vi "Launch uService.vi"(4 "Highlander?":bool, 6 "uService ID":string, 8 "error in (no error)":errorcluster, 9 "GUI?":bool, 10 "uService Class Name":string, 11 "Guardian in":refnum<class "Guardian.lvclass">) -> (0 "error out":errorcluster, 3 "Guardian out":refnum<class "Guardian.lvclass">)   [LabVIEW 2026, in "TALOS.lvlib" / "Guardian.lvlib" / "Guardian.lvclass"]
doc: "This VI get called everytime a uService has to be launched. The optional uService ID input is needed if a different name is wanted for a specific uService, otherwise the class name is used (useful when launching more than an instance of a uService, for example)."
uses:
  Guardian.lvclass
  C:/LabVIEW Code/TALOS/talos/Ancestor/Ancestor/Ancestor.lvclass
  C:/LabVIEW Code/TALOS/builds/Actor Framework PPL/Actor Framework.lvlibp/1abvi3w/vi.lib/ActorFramework/Actor/Actor.lvclass
  Classes/uService List/uService Properties.ctl
  builds/Actor Framework PPL/Actor Framework.lvlibp/1abvi3w/vi.lib/ActorFramework/Message Enqueuer/Message Enqueuer.lvclass
  Ancestor/Ancestor/Ancestor.lvclass/Ancestor.ctl
  Classes/uService List/uService List.lvclass/uService List.ctl
  Guardian Messages/Broadcast to Guardians Msg/Broadcast to Guardians Msg.lvclass/Broadcast to Guardians Msg.ctl
  Guardian.lvclass/Guardian.ctl
  Ancestor/Ancestor/Write Distr uS Map ref.vi
  Ancestor/Ancestor/Read ID.vi
  Ancestor/Ancestor/Read Distr uS Map ref.vi
  Support VIs/Generate Error.vi
  FGV/Error Memory/Get Error Description.vi
  Support VIs/Get PC name.vi
  Support VIs/Get Class Name.vi
  <vilib>/Utility/error.llb/Clear Errors.vi
  FGV/Error Memory/Error Memory Core.vi
  <vilib>/AdvancedString/Delimited String to 1D String Array.vi
  <vilib>/AdvancedString/Delimited String to 1D String Array (string).vi
  Support VIs/Circus Root Path.vi
  FGV/Error Memory/Error Crt Lvl checker.vi
  FGV/Error Memory/Error Memory Core.vi/40c8088d-b597-4017-91af-faa98e00292e.vi
  FGV/Error Memory/Error Memory Core.vi/d4a3ab98-063c-4e44-b43d-fbdcfe6c2be2.vi
  Father of all uServices/Father of all uServices/Father of all uServices.lvclass
  builds/Actor Framework PPL/Actor Framework.lvlibp/1abvi3w/vi.lib/ActorFramework/Message Enqueuer/Enqueue.vi
  Support VIs/Global Memory.vi
  <vilib>/Utility/LVClass/Get LV Class Name.vi
  Support VIs/Is in Packed Library.vi
  Support VIs/TALOS Root path.vi
  Support VIs/Read CSV worksheet.vi
  Support VIs/Global Constants.vi
  <vilib>/Utility/error.llb/General Error Handler.vi
  Support VIs/Error Log.vi
  Classes/Distributed uService Map/Distributed uService Map.lvclass
  Classes/uService List/uService List.lvclass
  Guardian Messages/Broadcast to Guardians Msg/Broadcast to Guardians Msg.lvclass
  Ancestor/Ancestor/Ancestor.lvclass
  <vilib>/Comparison/Equal/Equal Functor/Equal Functor.lvclass
  builds/Actor Framework PPL/Actor Framework.lvlibp/1abvi3w/vi.lib/ActorFramework/Actor/Actor.lvclass
  TALOS.lvlib
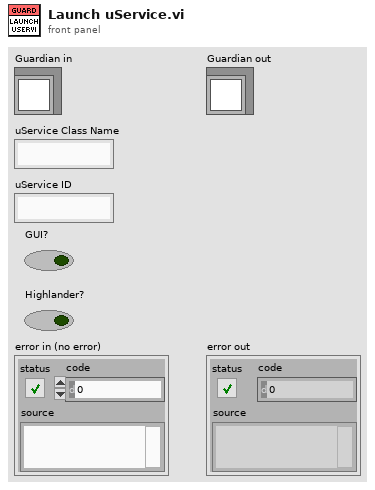
[diagram p1: front panel]
types:
  T1 = typedef "TALOS.lvlib/Classes.lvlib/uService List.lvclass/uService Properties.ctl" = cluster{"uService Queue":refnum<class "Message Enqueuer.lvclass">, "Last Pat":timestamp, "Online":bool, "Vi Ref":refnum<vi>, "Class name":string, "GUI":bool, "FP Items Refs Map":map{string, refnum<vi>}, "Remote GUI":bool, "Remote Window":refnum<vi>}
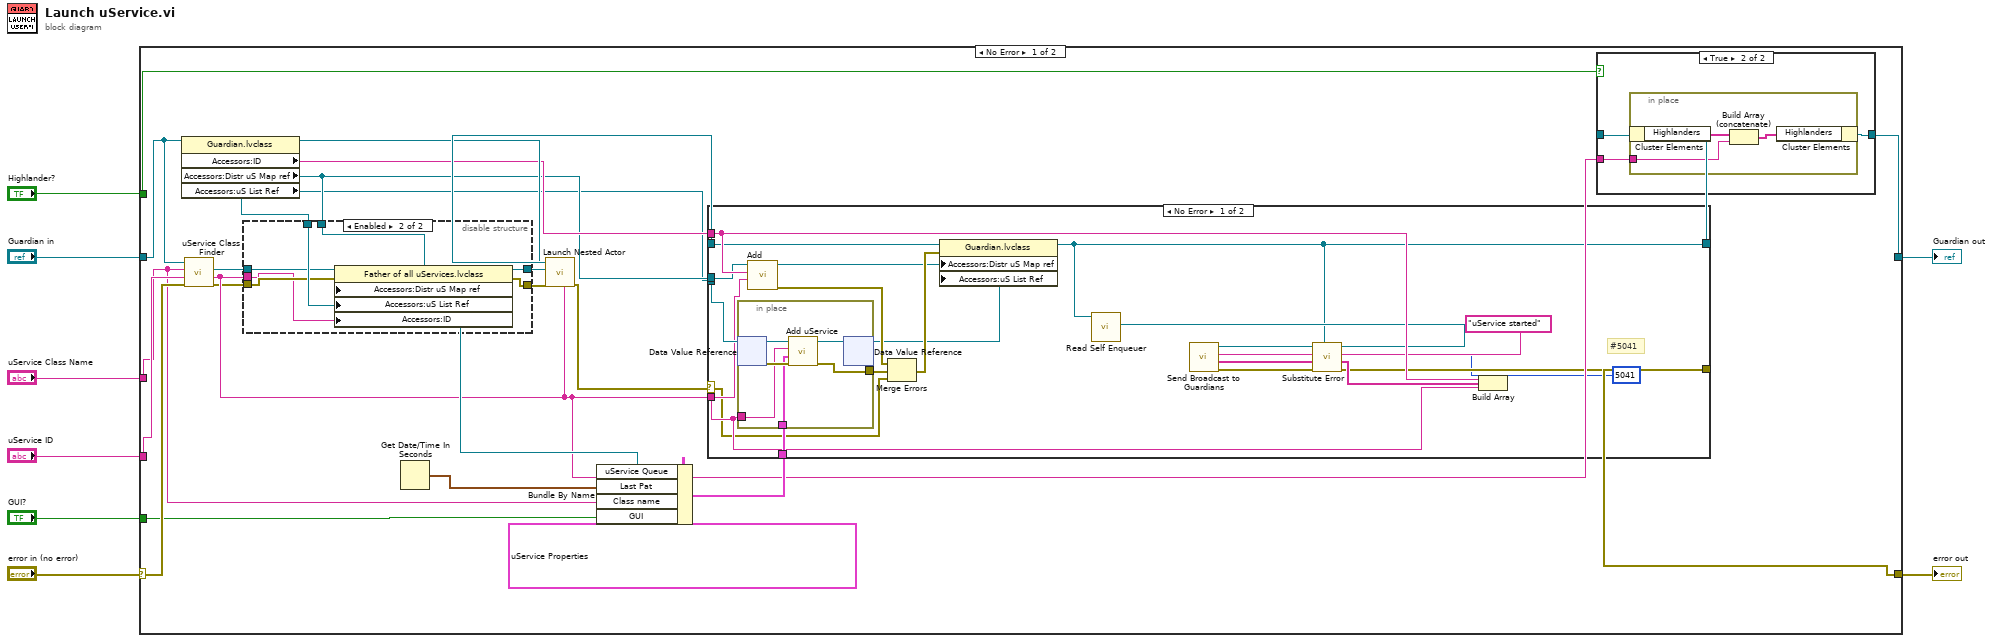
[diagram p0: block diagram]
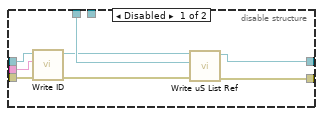
[diagram p2: hidden frame]
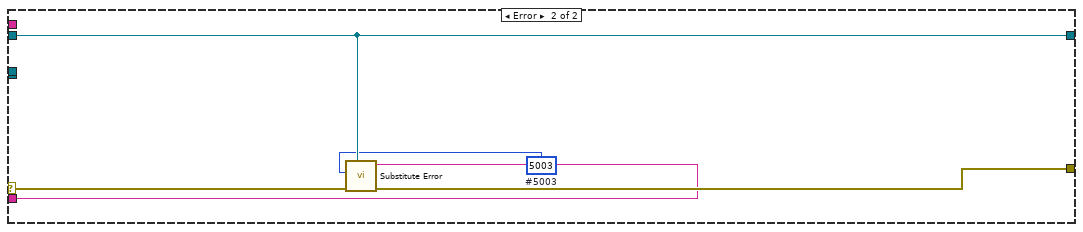
[diagram p3: hidden frame]
diagram:
  n1 = case shown="No Error" "error in (no error)" {
    selector: "error in (no error)" -> [w32 w85]
    tunnel: "Guardian in" -> [w24 w86]
    tunnel: "uService Class Name" -> [w23 _]
    tunnel: [w22 w85] -> w5
    tunnel: [w18 w86] -> w4
    tunnel: "GUI?" -> [w29 _]
    tunnel: "uService ID" -> [w25 _]
    tunnel: "Highlander?" -> [w20 _]
    frame No Error {
      n2 = property class="Guardian.lvclass"(reference=w24) -> (reference out=w16:refnum<class "Guardian.lvclass">, "Accessors:ID"=w15:string, "Accessors:Distr uS Map ref"=w14:refnum<data-value>, "Accessors:uS List Ref"=w13:refnum<data-value>)  [unwired: 1 in, 1 out]
      n3 = call "uService Class Finder.vi"("error in (no error)"=w32, "uService ID in"=w25, "uService Class name"=w23, "Guardian in"=w24) -> ("error out"=w11:errorcluster, "uService ID out"=w19:string, "uService out"=w10:refnum<class "Father of all uServices.lvclass">)  [unwired: 4 in, 1 out]
      n4 = disable-structure shown="Enabled" {
        disable-tunnel: w11 -> [w35 w46]
        disable-tunnel: [w39 w42] -> w12
        disable-tunnel: [w40 w41] -> w9
        disable-tunnel: w10 -> [w34 w45]
        disable-tunnel: w19 -> [w33 w44]
        disable-tunnel: w13 -> [w38 w47]
        disable-tunnel: w14 -> [_ w43]
        frame Disabled {
          n5 = call "Write ID.vi"("error in (no error)"=w35, "ID"=w33, "Ancestor in"=w34) -> ("error out"=w37:errorcluster, "Ancestor out"=w36:refnum<class "Father of all uServices.lvclass">)  [unwired: 7 in]
          n6 = call "Write uS List Ref.vi"("error in (no error)"=w37, "uS List Ref"=w38, "Ancestor in"=w36) -> ("error out"=w40:errorcluster, "Ancestor out"=w39:refnum<class "Father of all uServices.lvclass">)  [unwired: 7 in]
        }
        frame Enabled {
          n7 = property class="Father of all uServices.lvclass"(reference=w45, error in=w46, "Accessors:Distr uS Map ref"=w43, "Accessors:uS List Ref"=w47, "Accessors:ID"=w44) -> (reference out=w42:refnum<class "Father of all uServices.lvclass">, error out=w41:errorcluster)
        }
      }
      n8 = Get Date/Time In Seconds() -> (seconds since 1Jan1904=w31:timestamp)
      n9 = call "Launch Nested Actor.vi"("Debug Alias"=w19, "error in (no error)"=w9, "Nested Actor"=w12, "Caller Actor in"=w16) -> ("error out"=w26:errorcluster, "Nested Actor's Enqueuer"=w30:refnum<class "Message Enqueuer.lvclass">, "Caller Actor out"=w28:refnum<class "Guardian.lvclass">)  [unwired: 5 in]
      n10 = Bundle By Name(cluster=T1 {"uService Queue"=refnum, "Last Pat"=timestamp(0 s since 1904-01-01), "Online"=FALSE, "Vi Ref"=refnum, "Class name"="", "GUI"=FALSE, "FP Items Refs Map"={}, "Remote GUI"=FALSE, "Remote Window"=refnum} ("uService Properties"), "uService Queue"=w30, "Last Pat"=w31, "Class name"=w23, "GUI"=w29) -> (w27:T1)
      n11 = case shown="No Error" w26 {
        selector: w26 -> [w53 w77]
        tunnel: w28 -> [w48 w75]
        tunnel: w13 -> [w66 _]
        tunnel: w27 -> [w65 _]
        tunnel: w19 -> [w60 w74]
        tunnel: [w56 w75] -> w21
        tunnel: [w58 w76] -> w22
        tunnel: w15 -> [w63 _]
        tunnel: w14 -> [w50 _]
        frame No Error {
          # "#5041"
          n12 = in-place {
            in-place-border: w65 -> [w70]
            in-place-border: w60 -> [w69]
            in-place-border: [w68] -> w54
            n13 = in-place-dvr #1(w66) -> (w71:refnum<class "uService List.lvclass">, w72:errorcluster)
            n14 = call "Add uService.vi"("error in (no error)"=w72, "uService Properties"=w70, "ID"=w69, "uService List in"=w71) -> ("error out"=w68:errorcluster, "uService List out"=w67:refnum<class "uService List.lvclass">)  [unwired: 6 in]
            n15 = in-place-dvr #1(w67) -> (w49:refnum<data-value>)  [unwired: 1 out]
          }
          n16 = call "Add.vi"("uService"=w60, "Guardian"=w63, "Distr uS Map ref in"=w50) -> ("error out"=w52:errorcluster, "Distr uS Map ref out"=w51:refnum<data-value>)  [unwired: 6 in, 1 out]
          n17 = Merge Errors(w52, w54, w53) -> (w55:errorcluster)
          n18 = property class="Guardian.lvclass"(reference=w48, error in=w55, "Accessors:Distr uS Map ref"=w51, "Accessors:uS List Ref"=w49) -> (reference out=w56:refnum<class "Guardian.lvclass">)  [unwired: 1 out]
          n19 = call "Read Self Enqueuer.vi"("Actor"=w56) -> ("Self Enqueuer"=w61:refnum<class "Message Enqueuer.lvclass">)  [unwired: 10 in]
          n20 = Build Array(w63, w60) -> (w64:string[])
          n21 = call "Send Broadcast to Guardians.vi"("Data"=w64, "Message"="uService started", "Message Enqueuer"=w61) -> ("error out"=w59:errorcluster)  [unwired: 7 in, 1 out]
          n22 = call "Substitute Error.vi"("LabVIEW Object"=w56, "error in (no error)"=w59, "Error Code"=5041) -> ("error out"=w58:errorcluster)  [unwired: 8 in]
        }
        frame Error {
          w73 = 5003  # #5003
          n23 = call "Substitute Error.vi"("LabVIEW Object"=w75, "error in (no error)"=w77, "Error Code"=w73, "Optional String"=w74) -> ("error out"=w76:errorcluster)  [unwired: 7 in]
        }
      }
      n24 = case shown="True" w20 {
        tunnel: w21 -> [w78 w81]
        tunnel: w19 -> [_ w80]
        tunnel: [w78 w79] -> w18
        frame False {
        }
        frame True {
          n25 = in-place {
            in-place-border: w80 -> [w83]
            n26 = in-place-cluster #2(w81) -> ("Highlanders"=w84:string[])
            n27 = Build Array (concatenate)(w84, w83) -> (w82:string[])
            n28 = in-place-cluster #2("Highlanders"=w82) -> (w79:refnum<class "Guardian.lvclass">)
          }
        }
      }
    }
    frame Error {
    }
  }
  "error out" <- w5
  "Guardian out" <- w4
